vi "Idle.vi"(8 "error in (no error)":errorcluster, 11 "SV B-M (Target) in":refnum<class "SV B-M (Target).lvclass">) -> (0 "error out":errorcluster, 2 "Next State":string, 3 "SV B-M (Target) out":refnum<class "SV B-M (Target).lvclass">)   [LabVIEW 2015, in "SV B-M (Target).lvclass"]
uses:
  SV B-M (Target).lvclass
  Type Defs/Stream Param Cluster.ctl
  Type Defs/Sequence Parameters.ctl
  Type Defs/Target Type.ctl
  Type Defs/Variable Data Type.ctl
  SV B-M (Target).lvclass/SV B-M (Target).ctl
  Command & Ack - Receive Command.vi
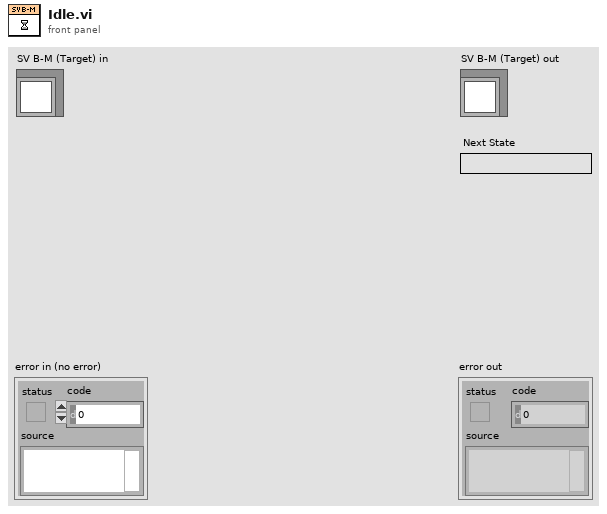
[diagram p1: front panel]
types:
  T1 = typedef "Stream Param Cluster.ctl" = cluster{"Seq Parameters":T2, "SV Library Info":cluster{"Lib Path":path, "Lib Size":u16}[]}
  T2 = typedef "Sequence Parameters.ctl" = cluster{"Test Name":string, "Target":T3, "Host IP Address":string, "Target IP Address":string, "Shared Variable Host":enum16{"Target", "Host"}, "Shared Variable Writer":enum16{"Target", "Host"}, "Variable Data Type":T4, "# of Variables per Library":u16, "Update Rate (Hz)":dbl, "Read Rate (Hz)":dbl, "Floor":u32, "Ceiling":u32, "Delta":u32}
  T3 = typedef "Target Type.ctl" = enum16{"cRIO-9012", "cRIO-9014", "cRIO-9022", "cRIO-9023", "cRIO-9024", "cRIO-9025", "cRIO-9068", "cRIO-9073", "cRIO-9074", "cRIO-9075", "cRIO-9076", "cRIO-9081", "cRIO-9082", "myRIO-1900", "myRIO-1950", "PXI-8101", "PXI-8115", "PXI-8119", "PXI-8820", "PXIe-8100", "PXIe-8101", "PXIe-8133", "PXIe-8135", "PXIe-8820", "sbRIO-9605", "sbRIO-9606", "sbRIO-9623", "sbRIO-9626", "sbRIO-9633", "sbRIO-9636", "Unlisted (Linux-RT)", "Unlisted (PharLap)", "Unlisted (VxWorks)", "Windows Target"}
  T4 = typedef "Variable Data Type.ctl" = enum16{"U8", "U16", "U32", "U64", "I8", "I16", "I32", "I64", "Single", "Double", "Boolean", "String"}
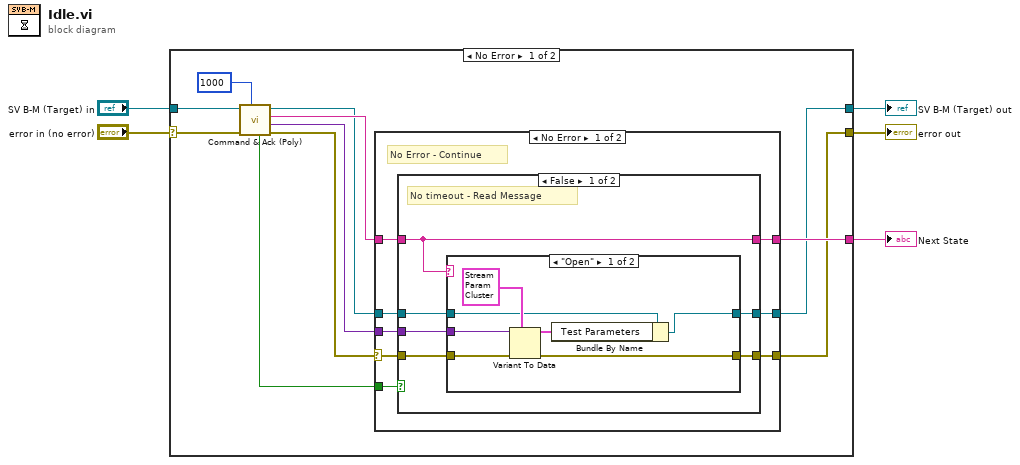
[diagram p0: block diagram]
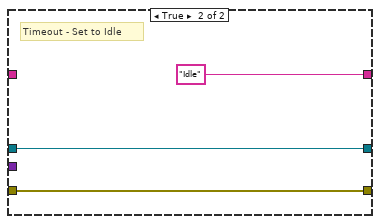
[diagram p3: hidden frame]
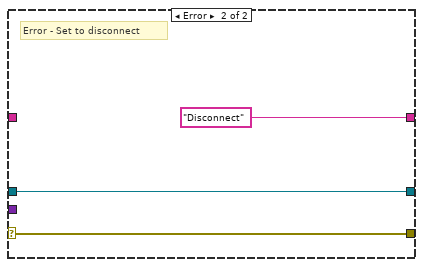
[diagram p4: hidden frame]
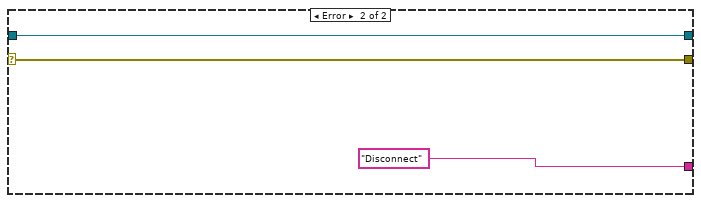
[diagram p5: hidden frame]
diagram:
  n1 = case shown="No Error" "error in (no error)" {
    selector: "error in (no error)" -> [w15 w48]
    tunnel: [w9 w48] -> w4
    tunnel: [w6 w47] -> w2
    tunnel: "SV B-M (Target) in" -> [w16 w47]
    tunnel: [w10 "Disconnect"] -> w1
    frame No Error {
      n2 = call-poly "Command & Ack (Poly).vi"("Timeout (-1)"=1000, "error in (no error)"=w15, "SV B-M (Target) in"=w16) -> ("error out"=w14:errorcluster, "Message Data"=w13:variant, "Message"=w12:string, "SV B-M (Target) out"=w7:refnum<class "SV B-M (Target).lvclass">, "Timeout?"=w11:bool)  [unwired: 4 in]
      n3 = case shown="No Error" w14 {
        selector: w14 -> [w21 w45]
        tunnel: w13 -> [w19 _]
        tunnel: w12 -> [w23 _]
        tunnel: w11 -> [w24 _]
        tunnel: [w22 "Disconnect"] -> w10
        tunnel: [w20 w45] -> w9
        tunnel: w7 -> [w18 w43]
        tunnel: [w17 w43] -> w6
        frame No Error {
          # "No Error - Continue"
          n4 = case shown="False" w24 {
            tunnel: w23 -> [w30 _]
            tunnel: [w30 "Idle" ("Message")] -> w22
            tunnel: [w25 w41] -> w20
            tunnel: w21 -> [w28 w41]
            tunnel: w19 -> [w29 _]
            tunnel: w18 -> [w27 w40]
            tunnel: [w26 w40] -> w17
            frame False {
              # "No timeout - Read Message"
              n5 = case shown="\"Open\"" w30 {
                tunnel: w29 -> [w37 _]
                tunnel: w28 -> [w36 w38]
                tunnel: w27 -> [w34 w39]
                tunnel: [w32 w39] -> w26
                tunnel: [w31 w38] -> w25
                frame "Open" {
                  n6 = Variant To Data(error in=w36, type=T1 {"Seq Parameters"={"Test Name"="Unique Test Name", "Target"=enum."cRIO-9012", "Host IP Address"="0.0.0.0", "Target IP Address"="0.0.0.0", "Shared Variable Host"=enum."Target", "Shared Variable Writer"=enum."Target", "Variable Data Type"=enum."Double", "# of Variables per Library"=500, "Update Rate (Hz)"=1.0, "Read Rate (Hz)"=1.0, "Floor"=500, "Ceiling"=5000, "Delta"=500}, "SV Library Info"=[]} ("Cluster"), Variant=w37) -> (data=w33:T1, error out=w31:errorcluster)
                  n7 = Bundle By Name(cluster=w34, "Test Parameters"=w33) -> (w32:refnum<class "SV B-M (Target).lvclass">)
                }
                frame Default {
                }
              }
            }
            frame True {
              # "Timeout - Set to Idle"
            }
          }
        }
        frame Error {
          # "Error - Set to disconnect"
        }
      }
    }
    frame Error {
    }
  }
  "error out" <- w4
  "SV B-M (Target) out" <- w2
  "Next State" <- w1
